vi "CAN BOOT Send App Data.vi"(5 "pCRC16":u16, 6 "DataLen":u16, 7 "pData":u8[](array[numeric])=array[4097 elements], 9 "NAD":u8, 10 "CANIndex":i32, 11 "DevHandle":i32) -> (1 "function return":i32, 2 "pCRC16 out":u16, 3 "pData out":u8[](array[numeric]))   [LabVIEW 2010, in "can_bootloader.lvlib"]
doc: "int WINAPI CAN_BOOT_SendAppData(int DevHandle,int CANIndex,unsigned char NAD,unsigned char *pData,unsigned short DataLen,unsigned short *pCRC16);"
uses:
  can_bootloader.lvlib
  USB2XXX/trunk/USB2XXX/USB2XXX/vs2010/Release/USB2XXX.dll
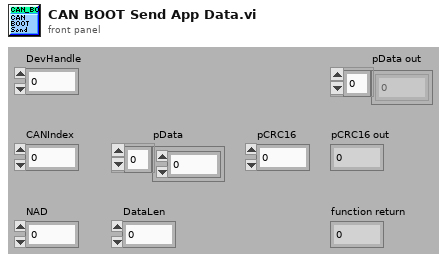
[diagram p1: front panel]
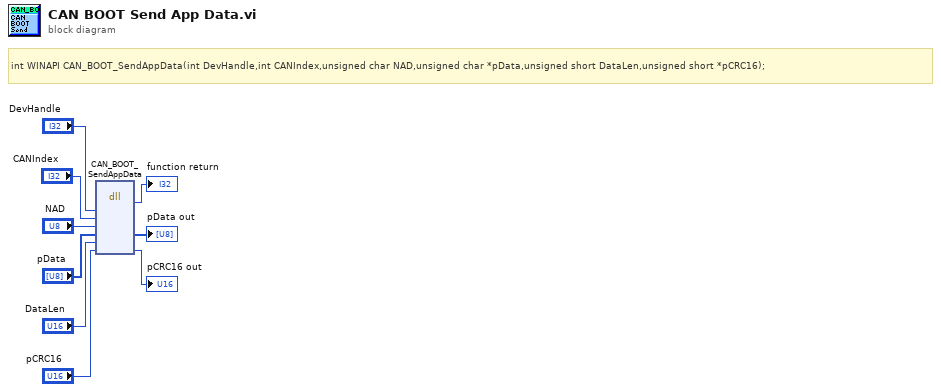
[diagram p0: block diagram]
diagram:
  # "int WINAPI CAN_BOOT_SendAppData(int DevHandle,int CANIndex,unsigned char NAD,unsigned char *pData,unsigned short DataLen,unsigned short *pCRC16);"
  n1 = dll-call lib="E:/OtherWork/STM32/USB2XXX/trunk/USB2XXX/USB2XXX/vs2010/Release/USB2XXX.*" fn="CAN_BOOT_SendAppData"("DevHandle"="DevHandle", "CANIndex"="CANIndex", "NAD"="NAD", "pData"="pData", "DataLen"="DataLen", "pCRC16"="pCRC16") -> (→"function return":i32, "pData"=→"pData out":u8[], "pCRC16"=→"pCRC16 out":u16)  [unwired: 7 in, 2 out]
